vi "FlipFlopSR.vi"(9 "Q":bool, 10 "R":bool, 11 "S":bool) -> (2 "Q\\":bool, 3 "Q+\nQ":bool)   [LabVIEW 2018]
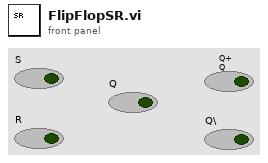
[diagram p1: front panel]
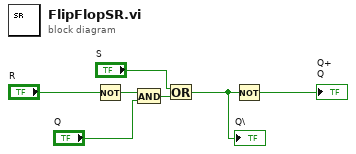
[diagram p0: block diagram]
diagram:
  n1 = Not(x="R") -> (.not. x?=w3:bool)
  n2 = And(x=w3, y="Q") -> (x .and. y?=w5:bool)
  n3 = Or(x="S", y=w5) -> (x .or. y?=w6:bool)
  "Q\\" <- w6
  n4 = Not(x=w6) -> (.not. x?=→"Q+\nQ":bool)
